vi "Sub_X_Scale_Change.vi"(7 "Target Scale":dbl, 11 "input":dbl[](array[numeric])) -> (3 "output":dbl[](array[numeric]))   [LabVIEW 2015]
panel:
  out "Unit of Index value":dbl
  out "Number of":dbl
  out "Number of addtional array = Target Scale - Number of Input":dbl
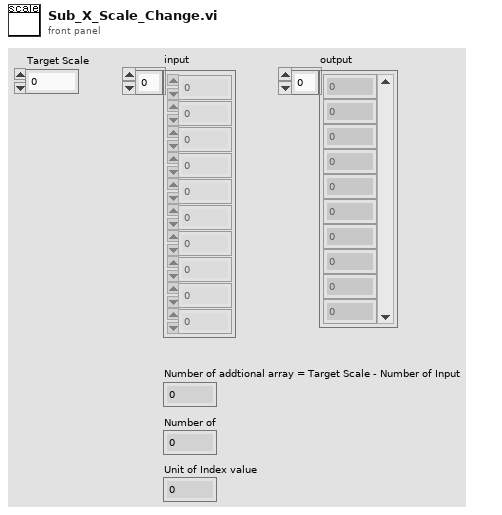
[diagram p1: front panel]
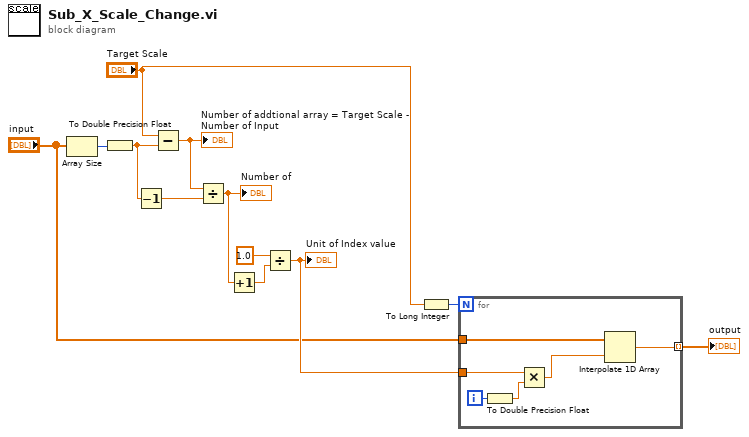
[diagram p0: block diagram]
diagram:
  n1 = Array Size(array="input") -> (size(s)=w12:i32)
  n2 = To Double Precision Float(number=w12) -> (double precision float=w6:dbl)
  n3 = Decrement(x=w6) -> (x-1=w11:dbl)
  n4 = Subtract(x="Target Scale", y=w6) -> (x-y=w10:dbl)
  "Number of addtional array = Target Scale - Number of Input" <- w10
  n5 = Divide(x=w10, y=w11) -> (x/y=w3:dbl)
  "Number of" <- w3
  n6 = Increment(x=w3) -> (x+1=w4:dbl)
  n7 = Divide(x=1.0, y=w4) -> (x/y=w8:dbl)
  "Unit of Index value" <- w8
  n8 = To Long Integer(number="Target Scale") -> (32bit integer=w9:i32)
  n9 = for {
    N: w9 -> [_]
    tunnel: w8 -> [w17]
    tunnel: "input" -> [w15]
    tunnel: [w14] -> w1 mode=indexing
    i -> [w18]
    n10 = To Double Precision Float(number=w18) -> (double precision float=w16:dbl)
    n11 = Multiply(x=w17, y=w16) -> (x*y=w13:dbl)
    n12 = Interpolate 1D Array(1:w13, 2:w15) -> (0:w14:dbl)
  }
  "output" <- w1
